vi "OverlayMessage.vi"(8 "error in (no error)":errorcluster, 10 "String in":string, 11 "UIRef":refnum<vi>) -> (0 "error out":errorcluster)   [LabVIEW 2024, in "GUI.lvlib" / "View.lvclass"]
uses:
  View.lvclass
  c52cbf22-949b-42b9-8f7f-037b2c70e477.vi
  View.lvclass/View.ctl
panel:
  out "String":string
types:
  T1 = typedef "LVRectTypeDef.ctl" = cluster{"Left":i16, "Top":i16, "Right":i16, "Bottom":i16}
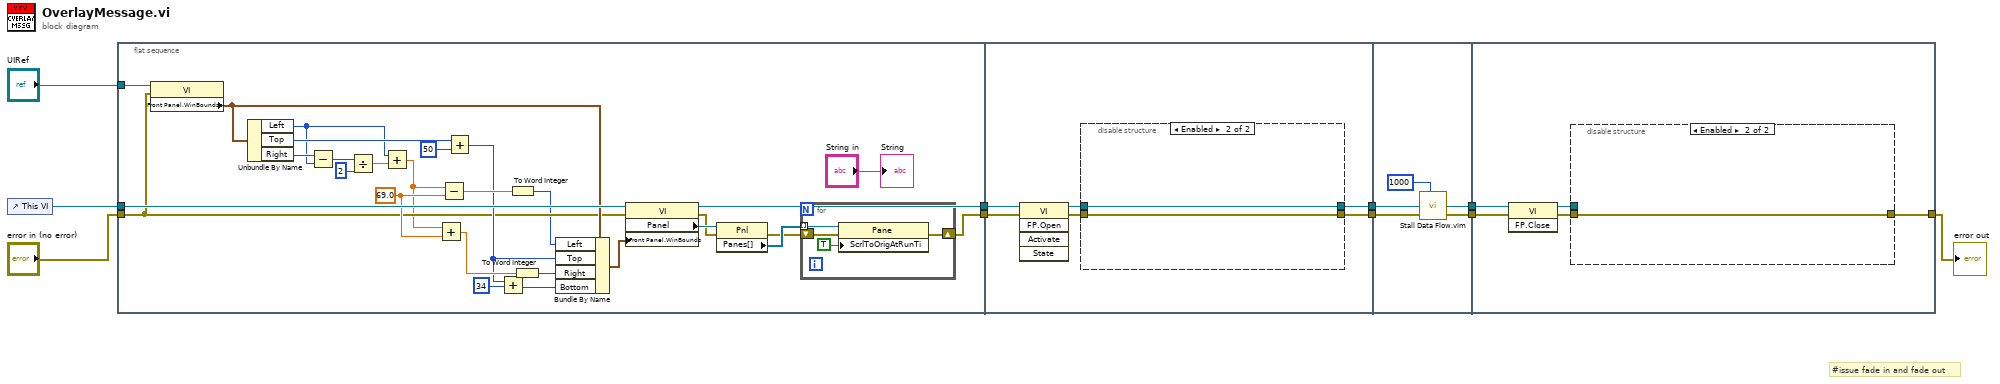
[diagram p0: block diagram]
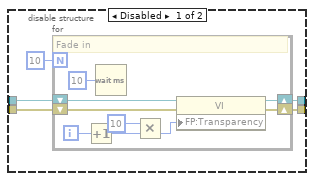
[diagram p2: hidden frame]
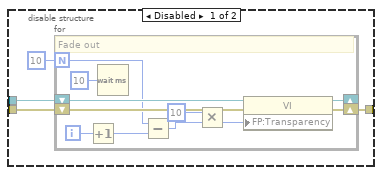
[diagram p3: hidden frame]
diagram:
  # "#issue fade in and fade out"
  n1 = control-ref of="This VI"() -> (w10:refnum<vi>)
  n2 = flat-sequence {
    tunnel: "error in (no error)" -> [w16]
    tunnel: w10 -> [w35]
    tunnel: [w33] -> w3
    tunnel: [w17] -> w2
    tunnel: "UIRef" -> [w37]
    tunnel: [w43] -> w8
    tunnel: [w44] -> w7
    tunnel: w3 -> [w48]
    tunnel: w2 -> [w47]
    tunnel: w8 -> [w67]
    tunnel: w7 -> [w68]
    tunnel: [w66] -> w6
    tunnel: [w68] -> w5
    tunnel: w6 -> [w73]
    tunnel: w5 -> [w72]
    tunnel: [w69] -> w4
    frame #0 {
      w27 = 69.0 ("y")
      n3 = property class="VI"(reference=w37, error in=w16) -> ("Front Panel.WinBounds"=w31:T1)  [unwired: 2 out]
      n4 = Unbundle By Name(w31) -> ("Left"=w14:i16, "Top"=w24:i16, "Right"=w30:i16)
      n5 = Subtract(x=w30, y=w14) -> (x-y=w29:i16)
      n6 = Divide(x=w29, y=i16 2) -> (x/y=w15:dbl)
      n7 = Add(x=w14, y=w15) -> (x+y=w13:dbl)
      n8 = Add(x=w13, y=w27) -> (x+y=w25:dbl)
      n9 = Subtract(x=w13, y=w27) -> (x-y=w26:dbl)
      n10 = Add(x=w24, y=i16 50) -> (x+y=w22:i16)
      n11 = Add(x=w22, y=i16 34) -> (x+y=w20:i16)
      n12 = To Word Integer(number=w26) -> (16bit integer=w12:i16)
      n13 = To Word Integer(number=w25) -> (16bit integer=w11:i16)
      n14 = Bundle By Name(cluster=w31, "Left"=w12, "Top"=w22, "Right"=w11, "Bottom"=w20) -> (w32:T1)
      n15 = property class="VI"(reference=w35, error in=w16, "Front Panel.WinBounds"=w32) -> (reference out=w33:refnum<vi>, error out=w19:errorcluster, "Panel"=w36:refnum<vi>)
      n16 = property class="Pnl"(reference=w36, error in=w19) -> (error out=w18:errorcluster, "Panes[]"=w34:refnum<vi>[])  [unwired: 1 out]
      n17 = for {
        tunnel: w34 -> [w42] mode=indexing
        shift-right: [w41] -> w17
        shift-left: w18 -> [w40]
        n18 = property class="Pane"(reference=w42, error in=w40, "ScrlToOrigAtRunTi"=TRUE ("Scroll To Origin At Run Time")) -> (error out=w41:errorcluster)  [unwired: 1 out]
      }
      "String" <- "String in"
    }
    frame #1 {
      n19 = invoke class="VI" method="FP.Open"(reference=w48, error in=w47) -> (reference out=w46:refnum<vi>, error out=w45:errorcluster)  [unwired: 3 in, 3 out]
      n20 = disable-structure shown="Enabled" {
        disable-tunnel: w46 -> [w52 w63]
        disable-tunnel: w45 -> [w51 w64]
        disable-tunnel: [w50 w64] -> w44
        disable-tunnel: [w49 w63] -> w43
        frame Disabled {
          n21 = for {
            N: 10 -> [_]
            shift-right: [w59] -> w49
            shift-left: w52 -> [w57]
            shift-right: [w58] -> w50
            shift-left: w51 -> [w56]
            i -> [w62]
            # "Fade in"
            n22 = Increment(x=w62) -> (x+1=w61:i32)
            n23 = Wait (ms)(milliseconds to wait=u32 10) -> ()  [unwired: 1 out]
            n24 = Multiply(x=10, y=w61) -> (x*y=w55:i32)
            n25 = property class="VI"(reference=w57, error in=w56, "FP:Transparency"=w55) -> (reference out=w59:refnum<vi>, error out=w58:errorcluster)
          }
        }
        frame Enabled {
        }
      }
    }
    frame #2 {
      n26 = call "Stall Data Flow.vim"("value in"=w67, "milliseconds to wait"=u32 1000) -> ("value out"=w66:refnum<vi>)  [unwired: 1 out]
    }
    frame #3 {
      n27 = invoke class="VI" method="FP.Close"(reference=w73, error in=w72) -> (reference out=w70:refnum<vi>, error out=w71:errorcluster)  [unwired: 1 in, 1 out]
      n28 = disable-structure shown="Enabled" {
        disable-tunnel: w71 -> [w77 w89]
        disable-tunnel: w70 -> [w76 _]
        disable-tunnel: [w74 w89] -> w69
        frame Disabled {
          n29 = for {
            N: 10 -> [w80]
            shift-right: [w86] -> _
            shift-left: w76 -> [w84]
            shift-right: [w85] -> w74
            shift-left: w77 -> [w83]
            i -> [w88]
            # "Fade out"
            n30 = Increment(x=w88) -> (x+1=w82:i32)
            n31 = Wait (ms)(milliseconds to wait=u32 10) -> ()  [unwired: 1 out]
            n32 = Subtract(x=w80, y=w82) -> (x-y=w81:i32)
            n33 = Multiply(x=10, y=w81) -> (x*y=w79:i32)
            n34 = property class="VI"(reference=w84, error in=w83, "FP:Transparency"=w79) -> (reference out=w86:refnum<vi>, error out=w85:errorcluster)
          }
        }
        frame Enabled {
        }
      }
    }
  }
  "error out" <- w4
